vi "Calibration.vi"(0 "Mode":T3, 5 "Calib file":path, 9 "Simulate/Run":T2) -> (14 "Calib const":string[][](array[string]), 16 "Coefficients":dbl[][](array[numeric]) format="%.2f", 19 "Status Out":T1)   [LabVIEW 2014]
uses:
  Anemometry Sub Vis/Calibration/Calib_mode.ctl
  Anemometry Sub Vis/Controls/User_Specific_mode.ctl
  Anemometry Sub Vis/Gen Trav/Multi_Run_Status.ctl
  Anemometry Sub Vis/Controls/Post_Process.ctl
  Anemometry Sub Vis/File/Setup_Filetype.ctl
  Anemometry Sub Vis/Controls/Setup.ctl
  Anemometry Sub Vis/Controls/Save_Data.ctl
  Anemometry Sub Vis/Controls/App_Global.ctl
  <vilib>/Analysis/baseanly.llb/Mean (DBL).vi
  Anemometry Sub Vis/Globals/Calib_global.vi
  Anemometry Sub Vis/Globals/Meas_global.vi
  Anemometry Sub Vis/Acquisition/PWA/PWAtasksGLOBAL.vi
  <vilib>/Analysis/NI_AALBase.lvlib
panel:
  in  "-ve Ref Values":bool
  out "String":string
  in  "polynomial order":i32=2 min=1 max=3 step=1
  out "Ref velocity":dbl[](array[numeric])=[2.4275346736, 2.4395664609, 2.453235235, 2.4247395837, 2.4277603784, 2.41169823, 2.4254144559, 2.424896502176921] format="%.3f"
  out "labels":string[](array[string])=["XW1 Volt", "XW2 Volt", "Entered Val", "Selector"]
  in  "Point selector 3":cluster{"Y":dbl, "X":dbl, "t/f":bool}[](array[cluster]) {"X" format="%#.2g"; "Y" format="%#.3f"}
  in  "n":dbl=0.45 format="%.4f"
  in  "Fixed n":bool=TRUE
  out "Sample of input signals":dbl[][](graph)
  in  "Sampling speeds":T4={"Samples/ch"=600, "Sample Rate/ch (Hz)"=100.0} {"Sample Rate/ch (Hz)" min=0; "Samples/ch" min=0 step=1}
  out "Calibration plot":cluster{cluster{dbl, dbl}[]}[](graph)
  in  "Point selector 4":T5(array[cluster]) {"Y2" format="%#.2f"; "X" format="%#.3f"; "Y" format="%#.2f"}
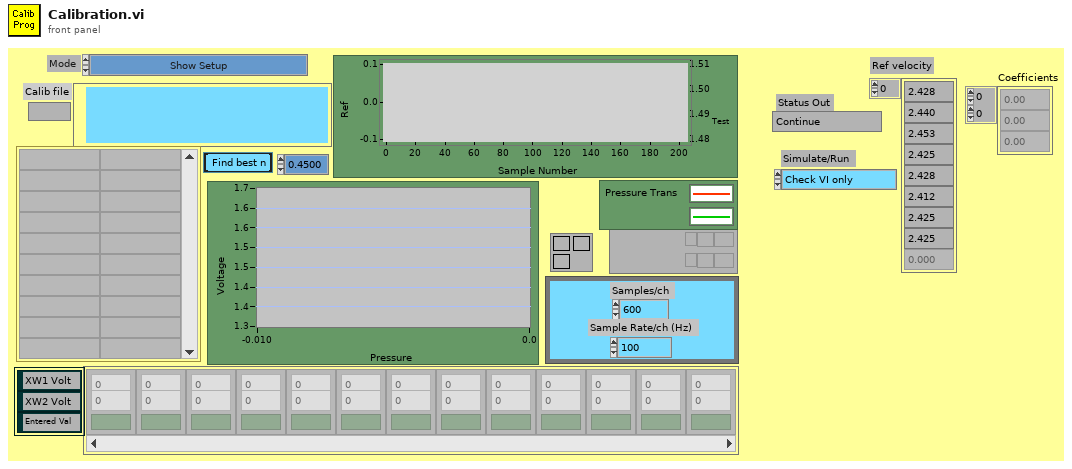
[diagram p1: front panel]
types:
  T1 = typedef "Multi_Run_Status.ctl" = enum16{"Continue", "Jump to Next Point", "Jump to Next Row", "Jump To Fall Back", "Terminate Run"}
  T2 = typedef "User_Specific_mode.ctl" = enum16{"Check VI only", "Run VI"}
  T3 = typedef "Calib_mode.ctl" = enum16{"Show Setup", "Take a New Calibration Point", "Refit Curve", "Setup Front Panel"}
  T4 = cluster{"Samples/ch":i32, "Sample Rate/ch (Hz)":sgl}
  T5 = cluster{"Y":dbl, "Y2":dbl, "X":dbl, "t/f":bool}[]
  T6 = typedef "Post_Process.ctl" = enum16{"Take New Data", "Post Process Raw Data File"}
  T7 = typedef "Setup_Filetype.ctl" = enum16{"Measurement Setups", "Calibration Setups", "General", "Results File Plotter Setups", "Speed Calib Tweaks"}
  T8 = typedef "Save_Data.ctl" = enum16{"Save No Data", "Save Data"}
  T9 = typedef "Setup.ctl" = enum16{"Run Program", "Show Setup", "Save Current Setup", "Setup Front Panel"}
  T10 = typedef "App_Global.ctl" = enum16{"Read Global", "Write to Global", "Initialise Array"}
  T11 = enum32{"existing file", "new file", "new or existing file", "existing dir", "new dir", "new or existing dir", "existing file (use LLBs)", "new file (use LLBs)", "new or existing file (use LLBs)", "new or existing file or directory (use LLBs)"}
  T12 = cluster{"Samples /ch":i32, "Sampling Rate /ch (Hz)":sgl}
  T13 = typedef "Cal_Inst_type.ctl" = enum16{"Propeller anemometer", "Pressure Transducer", "Hot wire", "Cross wire velocity", "Cross wire angle", "Generic Linear", "Generic Polynomial", "Generic BackPoly", "Fast FID", "Thermocouple", "Cold wire", "Pulsed Wire"}
  T14 = typedef "Ref_Inst_type.ctl" = enum16{"Propellor anemometer", "Pressure Transducer", "Raw voltage", "Pitot-static tube", "Preston tube", "Generic Linear", "Generic Polynomial", "Thermocouple", "LDA", "Enter Value", "ADAM Channel"}
  T15 = cluster{"2nd Ref type":T14, "2nd inst present":bool}
  T16 = typedef "Analysis_info_cluster.ctl" = cluster{"Colour":u32, "Inst type":T17, "Inst name":string, "Symbol":string, "Code name":string, "Extra Info":string, "Inst Array":T18, "Extra Titles":string[], "Extra Values":string[], "U":dbl, "u^2":dbl, "u^3":dbl, "u^4":dbl, "Skew_u":dbl, "Kurt_u":dbl, "Sd Error in Mean":dbl, "% u'/U":dbl, "X":dbl, "Y":dbl, "Z":dbl, "Timescale integral to 25%":dbl, "Sd Error in Variance":dbl, "Calib File":path, "Calib Constants":dbl[], "Output Position":bool, "Full Stats":bool, "Av Sampling Rate":dbl, "Av No of Samples":dbl, "Total Meas Time (s)":dbl, "ADAM Ch Name":string}
  T17 = typedef "Inst_type.ctl" = enum16{"Propeller anemometer", "Raw voltage", "Pressure Transducer", "Pitot-static tube", "Preston tube", "Hot wire", "Cross wire 1", "Cross wire 2", "Generic Linear", "Generic Polynomial", "Generic BackPoly", "Fast FID", "Thermocouple", "Cold wire", "Pulsed Wire", "LDA Vel", "LDA Tran time", "LDA Arr time", "Microphone"}
  T18 = typedef "Instrument_Array.ctl" = enum16{"PWA", "LDA", "Analogue"}
  T19 = typedef "Time_Trace_Cluster.ctl" = cluster{"Weighting":dbl[], "Time (s)":dbl[], "Voltage":dbl[], "Eng Values":dbl[]}
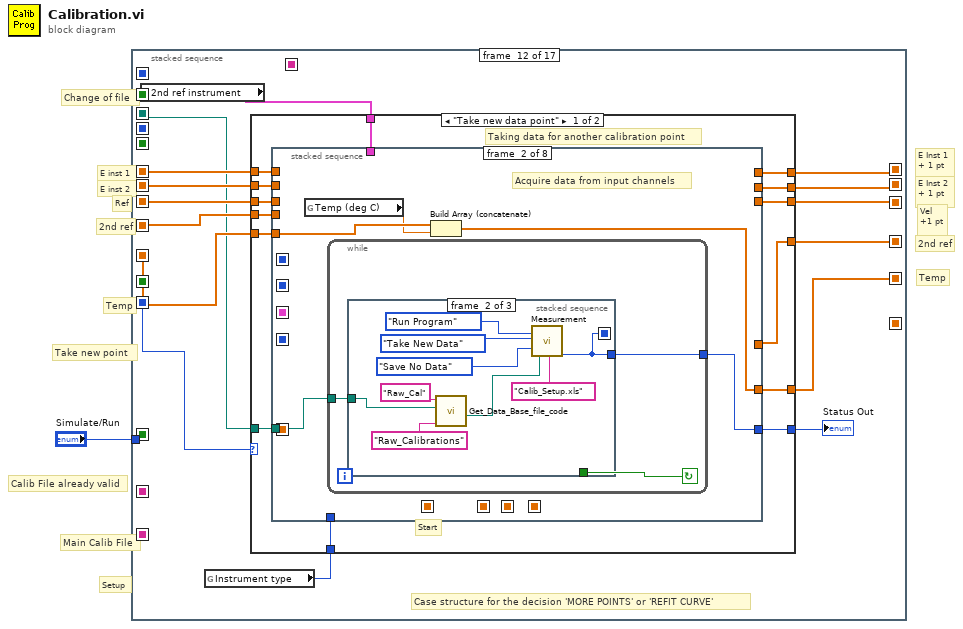
[diagram p0: block diagram]
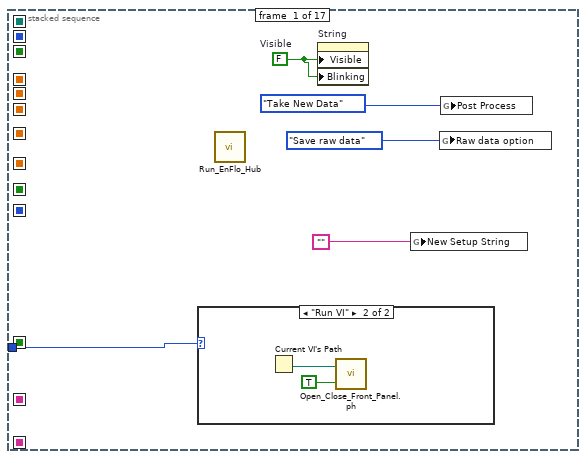
[diagram p2: hidden frame]
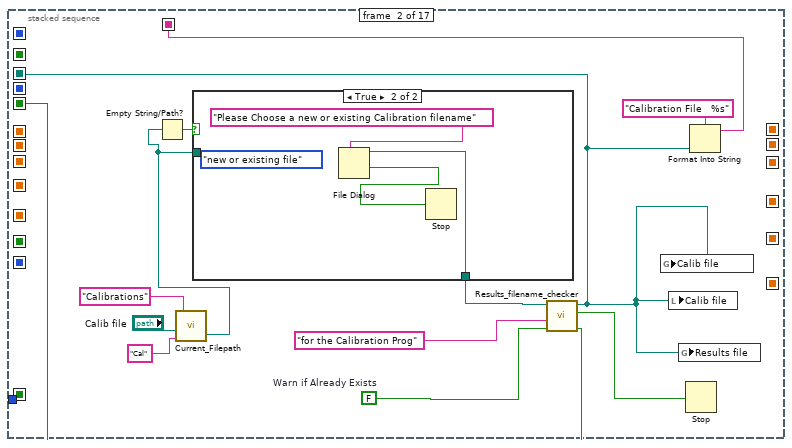
[diagram p4: hidden frame]
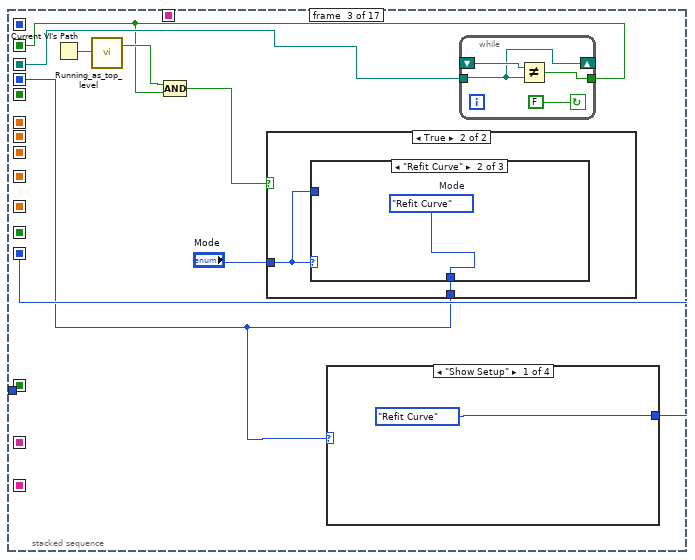
[diagram p6: hidden frame]
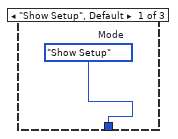
[diagram p8: hidden frame]
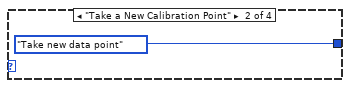
[diagram p10: hidden frame]
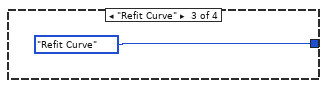
[diagram p11: hidden frame]
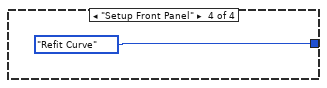
[diagram p12: hidden frame]
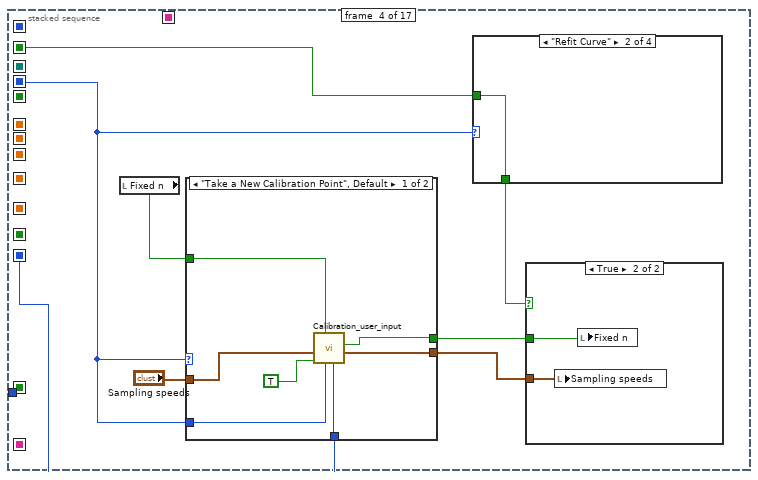
[diagram p13: hidden frame]
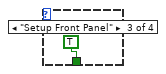
[diagram p15: hidden frame]
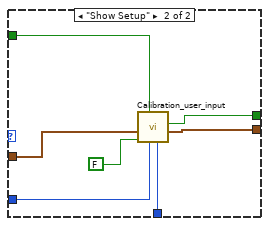
[diagram p18: hidden frame]
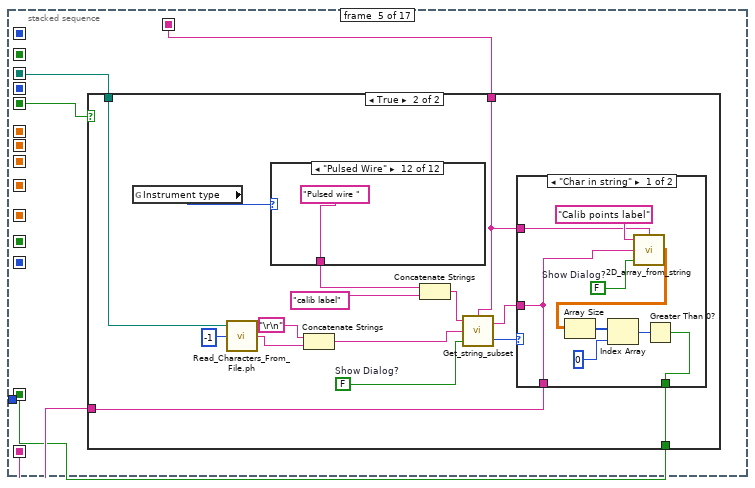
[diagram p19: hidden frame]
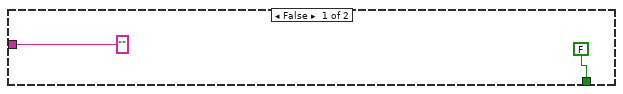
[diagram p20: hidden frame]
diagram:
  # "Change of file"
  # "Take new point"
  # "Calib File already valid"
  # "Main Calib File"
  # "Temp"
  # "Temp"
  # "Setup"
  # "E inst 1"
  # "Ref"
  # "E Inst 1\n+ 1 pt"
  # "Vel\n+1 pt"
  # "E inst 2"
  # "E Inst 2\n+ 1 pt"
  # "2nd ref"
  # "2nd ref"
  n1 = stacked-sequence {
    seq-local: [_ _ _ _ _ _ _ _ _ _ _ w490 _ _ _ _ _] -> [_ _ _ _ _ _ _ _ _ _ _ _ w690 _ _ _ _]
    seq-local: [_ _ _ _ _ _ _ _ _ _ _ w489 _ _ _ _ _] -> [_ _ _ _ _ _ _ _ _ _ _ _ w693 _ _ w756 _]
    seq-local: [_ _ _ _ _ _ _ w377 _ _ _ _ _ _ _ _ _] -> [_ _ _ _ _ _ _ _ _ _ _ w492 _ _ _ _ _]
    seq-local: [_ _ _ _ _ _ _ w376 _ _ _ _ _ _ _ _ _] -> [_ _ _ _ _ _ _ _ _ _ _ w491 _ _ _ _ _]
    seq-local: [_ _ _ _ _ _ _ w375 _ _ _ _ _ _ _ _ _] -> [_ _ _ _ _ _ _ _ _ _ _ w487 _ _ _ _ _]
    seq-local: [_ _ _ _ _ _ _ _ _ _ _ w488 _ _ _ _ _] -> [_ _ _ _ _ _ _ _ _ _ _ _ w692 _ _ _ _]
    seq-local: [_ _ _ _ _ _ _ w374 _ _ _ _ _ _ _ _ _] -> [_ _ _ _ _ _ _ _ _ _ _ w486 _ _ _ _ _]
    seq-local: [_ _ _ _ _ _ _ _ _ _ _ w485 _ _ _ _ _] -> [_ _ _ _ _ _ _ _ _ _ _ _ w687 _ _ _ _]
    seq-local: [_ _ _ _ w79 _ _ _ _ _ _ _ _ _ _ _ _] -> [_ _ _ _ _ _ _ w363 _ _ _ _ _ _ _ _ _]
    seq-local: [_ _ _ _ w80 _ _ _ _ _ _ _ _ _ _ _ _] -> [_ _ _ _ _ _ _ w364 _ _ _ _ _ _ _ _ _]
    seq-local: [_ _ _ _ _ _ _ _ _ _ w465 _ _ _ _ _ _] -> [_ _ _ _ _ _ _ _ _ _ _ _ _ _ w734 _ _]
    seq-local: [_ _ _ _ _ _ _ _ _ _ _ w483 _ _ _ _ _] -> [_ _ _ _ _ _ _ _ _ _ _ _ w691 _ _ _ _]
    seq-local: [_ _ _ _ _ _ _ w373 _ _ _ _ _ _ _ _ _] -> [_ _ _ _ _ _ _ _ _ _ _ w482 _ _ _ _ _]
    seq-local: [_ w14 _ _ _ _ _ _ _ _ _ _ _ _ _ _ _] -> [_ _ w30 _ w78 _ _ _ _ _ w466 w480 _ w716 w743 w757 _]
    seq-local: [_ w19 _ _ _ _ _ _ _ _ _ _ _ _ _ _ _] -> [_ _ _ _ w77 _ _ _ w406 _ _ _ _ _ _ _ _]
    seq-local: [_ _ w33 _ _ _ _ _ _ _ _ _ _ _ _ _ _] -> [_ _ _ w51 _ _ _ _ _ _ _ w479 _ _ _ w758 _]
    seq-local: [_ _ w26 _ _ _ _ _ _ _ _ _ _ _ _ _ _] -> [_ _ _ w50 _ _ _ _ _ w423 _ _ _ _ _ _ w800]
    seq-local: [_ _ _ _ _ _ _ w365 _ _ _ _ _ _ _ _ _] -> [_ _ _ _ _ _ _ _ w404 _ _ _ _ _ _ _ _]
    seq-local: [_ _ _ _ _ _ _ _ _ _ _ _ w688 _ _ _ _] -> [_ _ _ _ _ _ _ _ _ _ _ _ _ w700 _ _ _]
    seq-local: [_ _ _ _ _ _ _ _ _ _ _ _ w686 _ _ _ _] -> [_ _ _ _ _ _ _ _ _ _ _ _ _ w715 _ _ _]
    seq-local: [_ _ w29 _ _ _ _ _ _ _ _ _ _ _ _ _ _] -> [_ _ _ w48 _ _ _ _ w403 _ _ _ _ _ _ _ _]
    seq-local: [_ w13 _ _ _ _ _ _ _ _ _ _ _ _ _ _ _] -> [_ _ _ _ w76 _ _ w358 _ _ _ _ _ _ _ _ _]
    tunnel: "Simulate/Run" -> [w5 _ _ _ _ _ _ _ _ _ _ _ _ _ _ _ _]
    frame #0 {
      w3 = FALSE  # Visible
      n2 = case shown="\"Run VI\"" w5 {
        frame "Check VI only" {
        }
        frame "Run VI" {
          n3 = Current VI's Path() -> (path=w7:path)
          n4 = call "Open_Close_Front_Panel.ph.vi"("Front Panel Window:Open"=TRUE, "VI path"=w7) -> ()  [unwired: 2 out]
        }
      }
      n5 = call "Run_EnFlo_Hub.vi"() -> ()  [unwired: 8 out]
      n6 = property on="String" class="Str"("Visible"=w3, "Blinking"=w3) -> ()  [unwired: 2 in, 2 out]
      n7 = global write "Calib_global.vi" "New Setup String"("") -> ()
      n8 = global write "Meas_global.vi" "Raw data option"(enum16{"Save raw data", "Raw data not saved"}."Save raw data" ("Raw data option")) -> ()
      n9 = global write "Meas_global.vi" "Post Process"(Post_Process."Take New Data" ("Post Process")) -> ()
    }
    frame #1 {
      w20 = FALSE  # Warn if Already Exists
      n10 = call "Current_Filepath.vi"("Short_Name"="Cal" ("Data Type"), "Filename in"="Calib file", "Data Type"="Calibrations") -> ("Filename Out"=w11:path)  [unwired: 1 in, 1 out]
      n11 = Empty String/Path?(string/path=w11) -> (empty?=w16:bool)
      n12 = case shown="True" w16 {
        tunnel: w11 -> [w22 _]
        tunnel: [w22 w24] -> w18
        frame False {
        }
        frame True {
          (unwired) T11."new or existing file" ("select mode (2)")
          n13 = File Dialog(7:"Please Choose a new or existing Calibration filename" ("Promp if not found")) -> (1:w23:bool, 3:w24:path)  [unwired: 1 in, 7 out]
          n14 = Stop(stop? (T)=w23) -> ()
        }
      }
      n15 = call "Results_filename_checker.vi"("Warn if Already Exists"=w20, "Comment"="for the Calibration Prog", "Results file"=w18) -> ("exists?"=w19:bool, "cancelled"=w17:bool, "Results file output"=w14:path)  [unwired: 2 in, 1 out]
      n16 = global write "Calib_global.vi" "Calib file"(w14) -> ()
      n17 = local write "Calib file"(w14) -> ()
      n18 = global write "Meas_global.vi" "Results file"(w14) -> ()
      n19 = Stop(stop? (T)=w17) -> ()
      n20 = Format Into String(format string="Calibration File   %s", w14) -> (resulting string=w13:string)  [unwired: 2 in, 1 out]
    }
    frame #2 {
      n21 = Current VI's Path() -> (path=w32:path)
      n22 = call "Running_as_top_level.vi"("Vi path name"=w32) -> ("Top Level"=w31:bool)  [unwired: 1 out]
      n23 = while {
        shift-right: [w42] -> _
        shift-left: _ -> [w43]
        tunnel: w30 -> [w42]
        tunnel: [w41] -> w29
        stop <- FALSE continue-if-true
        n24 = Not Equal?(x=w43, y=w42) -> (x != y?=w41:bool)
      }
      n25 = Compound Arithmetic op=AND(w31, w29) -> (w28:bool)
      n26 = case shown="True" w28 {
        tunnel: "Mode" -> [w34 w35]
        tunnel: [w34 w36] -> w26
        frame False {
        }
        frame True {
          n27 = case shown="\"Refit Curve\"" w35 {
            tunnel: [w37 w38 w39] -> w36
            tunnel: w35 -> [_ _ w39]
            frame "Show Setup", Default {
              w37 = Calib_mode."Show Setup"  # Mode
            }
            frame "Refit Curve" {
              w38 = Calib_mode."Refit Curve"  # Mode
            }
            frame "Setup Front Panel" {
            }
          }
        }
      }
      n28 = case shown="\"Show Setup\"" w26 {
        tunnel: [enum16{"Take new data point", "Refit Curve"}."Refit Curve" ("data mode") enum16{"Take new data point", "Refit Curve"}."Take new data point" ("data mode") enum16{"Take new data point", "Refit Curve"}."Refit Curve" ("data mode") enum16{"Take new data point", "Refit Curve"}."Refit Curve" ("data mode")] -> w33
        frame "Show Setup" {
        }
        frame "Take a New Calibration Point" {
        }
        frame "Refit Curve" {
        }
        frame "Setup Front Panel" {
        }
      }
    }
    frame #3 {
      n29 = local read "Fixed n"() -> (w53:bool)
      n30 = case shown="\"Take a New Calibration Point\", Default" w50 {
        tunnel: "Sampling speeds" -> [w68 w75]
        tunnel: w50 -> [w66 w73]
        tunnel: w51 -> [w65 w72]
        tunnel: [w64 w71] -> w54
        tunnel: w53 -> [w62 w70]
        tunnel: [w63 w69] -> w52
        frame "Take a New Calibration Point", Default {
          n31 = call "Calibration_user_input.vi"("data mode"=w65, "Mode"=w66, "Fixed n"=w62, "OK"=TRUE, "Sampling speeds"=w68) -> ("Sampling speeds Output"=w64:T12, "Fixed n out"=w63:bool)  [unwired: 2 in, 3 out]
        }
        frame "Show Setup" {
          n32 = call "Calibration_user_input.vi"("data mode"=w72, "Mode"=w73, "Fixed n"=w70, "OK"=FALSE, "Sampling speeds"=w75) -> ("Sampling speeds Output"=w71:T12, "Fixed n out"=w69:bool)  [unwired: 5 out]
        }
      }
      n33 = case shown="\"Refit Curve\"" w50 {
        tunnel: [w56 w57 TRUE w59] -> w49
        tunnel: w48 -> [w56 w57 _ w59]
        frame "Show Setup" {
        }
        frame "Refit Curve" {
        }
        frame "Setup Front Panel" {
        }
        frame "Take a New Calibration Point" {
        }
      }
      n34 = case shown="True" w49 {
        tunnel: w54 -> [_ w61]
        tunnel: w52 -> [_ w60]
        frame False {
        }
        frame True {
          n35 = local write "Sampling speeds"(w61) -> ()
          n36 = local write "Fixed n"(w60) -> ()
        }
      }
    }
    frame #4 {
      n37 = case shown="True" w77 {
        tunnel: ["" ("Output string") w97] -> w80
        tunnel: [FALSE w96] -> w79
        tunnel: w78 -> [_ w88]
        tunnel: w76 -> [_ w83]
        frame False {
        }
        frame True {
          w87 = FALSE  # Show Dialog?
          n38 = global read "Calib_global.vi" "Instrument type"() -> (w91:T13)
          n39 = call "Read_Characters_From_File.ph.vi"("file path (dialog if empty)"=w88, "number of characters (all:-1)"=-1) -> ("character string"=w85:string)  [unwired: 7 out]
          n40 = case shown="\"Pulsed Wire\"" w91 {
            tunnel: ["Prop " "Mano " "HW " "Cross wire velocity " "Cross wire angle " "Generic Inst " "Generic Polynomial " "Generic BackPoly " "Fast FID " "Thermocouple " "Cold wire " "Pulsed wire "] -> w92
            frame "Propeller anemometer" {
            }
            frame "Pressure Transducer" {
            }
            frame "Hot wire" {
            }
            frame "Cross wire velocity" {
            }
            frame "Cross wire angle" {
            }
            frame "Generic Linear" {
            }
            frame "Generic Polynomial" {
            }
            frame "Generic BackPoly" {
            }
            frame "Fast FID" {
            }
            frame "Thermocouple" {
            }
            frame "Cold wire" {
            }
            frame "Pulsed Wire" {
            }
          }
          n41 = Concatenate Strings("\r\n", w85) -> (w84:string)
          n42 = Concatenate Strings(w92, "calib label") -> (w93:string)
          n43 = call "Get_string_subset.vi"("String Name"=w83, "Show Dialog?"=w87, "String to split"=w84, "File Label"=w93) -> ("Status"=w90:enum16{"Char in string", "Char not in string"}, "Output string"=w89:string)
          n44 = case shown="\"Char in string\"" w90 {
            tunnel: w89 -> [w116 _]
            tunnel: [w116 ""] -> w97
            tunnel: [w111 FALSE] -> w96
            tunnel: w83 -> [w110 _]
            frame "Char in string" {
              w117 = FALSE  # Show Dialog?
              n45 = call "2D_array_from_string.vi"("String Name"=w110, "Show Dialog?"=w117, "Input string"=w116, "Array title"="Calib points label") -> ("2D data array"=w115:dbl[][])
              n46 = Array Size(array=w115) -> (size(s)=w114:i32[])
              n47 = Index Array(array=w114, index=0 ("Index")) -> (element=w112:i32)
              n48 = Greater Than 0?(x=w112) -> (x > 0?=w111:bool)
            }
            frame "Char not in string" {
            }
          }
        }
      }
    }
    frame #5 {
      w123 = ""
      n49 = global read "Calib_global.vi" "2nd ref instrument"() -> (w130:T15)
      n50 = global read "Calib_global.vi" "Ref Instrument type"() -> (w131:T14)
      n51 = Unbundle By Name(w130) -> ("2nd Ref type"=w128:T14, "2nd inst present"=w129:bool)
      n52 = global read "Calib_global.vi" "Instrument type"() -> (w134:T13)
      n53 = case shown="\"Propellor anemometer\"" w131 {
        tunnel: [w160 w163 w167 w169 w172 w175 w178 w181 w184 string[] [] string[] []] -> w127
        tunnel: [FALSE FALSE FALSE FALSE TRUE FALSE FALSE FALSE FALSE FALSE FALSE] -> w122
        frame "Propellor anemometer" {
          n54 = Build Array("Prop Velocity") -> (w160:string[])
        }
        frame "Pressure Transducer" {
          n55 = Build Array("Pressure Trans") -> (w163:string[])
        }
        frame "Raw voltage" {
          n56 = Build Array("Raw Voltage") -> (w167:string[])
        }
        frame "Pitot-static tube" {
          n57 = Build Array("Pitot Vel") -> (w169:string[])
        }
        frame "Preston tube" {
          n58 = Build Array("Shear stress") -> (w172:string[])
        }
        frame "Generic Linear" {
          n59 = Build Array("Gen Lin") -> (w175:string[])
        }
        frame "Generic Polynomial" {
          n60 = Build Array("Gen Poly") -> (w178:string[])
        }
        frame "Thermocouple" {
          n61 = Build Array("Thermo") -> (w181:string[])
        }
        frame "LDA" {
          n62 = Build Array("LDA Vel") -> (w184:string[])
        }
        frame "Enter Value" {
        }
        frame "ADAM Channel" {
        }
      }
      n63 = case shown="True" w129 {
        tunnel: w128 -> [_ w137]
        tunnel: [w136 w138] -> w125
        tunnel: w127 -> [w136 _]
        frame False {
        }
        frame True {
          n64 = case shown="\"Propellor anemometer\"" w137 {
            tunnel: [w139 w141 w144 w145 w147 w149 w151 w153 w155 string[] [] string[] []] -> w138
            frame "Propellor anemometer" {
              n65 = Build Array("Prop Velocity") -> (w139:string[])
            }
            frame "Pressure Transducer" {
              n66 = Build Array("Pressure Trans") -> (w141:string[])
            }
            frame "Raw voltage" {
              n67 = Build Array("Raw Voltage") -> (w144:string[])
            }
            frame "Pitot-static tube" {
              n68 = Build Array("Pitot Vel") -> (w145:string[])
            }
            frame "Preston tube" {
              n69 = Build Array("Shear stress") -> (w147:string[])
            }
            frame "Generic Linear" {
              n70 = Build Array("Gen Lin") -> (w149:string[])
            }
            frame "Generic Polynomial" {
              n71 = Build Array("Gen Poly") -> (w151:string[])
            }
            frame "Thermocouple" {
              n72 = Build Array("Thermo") -> (w153:string[])
            }
            frame "LDA" {
              n73 = Build Array("LDA Vel") -> (w155:string[])
            }
            frame "Enter Value" {
            }
            frame "ADAM Channel" {
            }
          }
        }
      }
      n74 = case shown="\"Pulsed Wire\"" w134 {
        tunnel: [w194 w198 w202 w206 w211 w216 w220 w224 w228 w232 w236 w241] -> w124
        tunnel: [FALSE FALSE FALSE FALSE FALSE FALSE TRUE TRUE FALSE FALSE TRUE TRUE] -> w126
        tunnel: [w192 w196 w200 w204 w209 w214 w218 w222 w226 w230 w234 FALSE] -> w121
        tunnel: w122 -> [w192 w196 w200 w204 w209 w214 w218 w222 w226 w230 w234 _]
        frame "Propeller anemometer" {
          n75 = Build Array("Prop Voltage") -> (w194:string[])
        }
        frame "Pressure Transducer" {
          n76 = Build Array("Pressure Trans") -> (w198:string[])
        }
        frame "Hot wire" {
          n77 = Build Array("HW Voltage") -> (w202:string[])
        }
        frame "Cross wire velocity" {
          n78 = Build Array("XW1 Voltage", "XW2 Voltage") -> (w206:string[])
        }
        frame "Cross wire angle" {
          n79 = Build Array("XW1 Voltage", "XW2 Voltage") -> (w211:string[])
        }
        frame "Generic Linear" {
          n80 = Build Array("Generic Voltage") -> (w216:string[])
        }
        frame "Generic Polynomial" {
          n81 = Build Array("Generic Voltage") -> (w220:string[])
        }
        frame "Generic BackPoly" {
          n82 = Build Array("Generic Voltage") -> (w224:string[])
        }
        frame "Fast FID" {
          n83 = Build Array("FF Voltage") -> (w228:string[])
        }
        frame "Thermocouple" {
          n84 = Build Array("Thermo Voltage") -> (w232:string[])
        }
        frame "Cold wire" {
          n85 = Build Array("CW Voltage") -> (w236:string[])
        }
        frame "Pulsed Wire" {
          n86 = local write "polynomial order"(3 ("polynomial order")) -> ()
          n87 = Build Array("PWA 1/TOF") -> (w241:string[])
        }
      }
      n88 = property on="polynomial order" class="DigNum (strict)"("Visible"=w126) -> ()  [unwired: 2 in, 2 out]
      n89 = Build Array (concatenate)(w125, w124, w123, w123, w123) -> (w132:string[])
      n90 = for {
        N: 3 -> [_]
        tunnel: w132 -> [w190] mode=indexing
        i -> [w191]
        n91 = property on="Sample of input signals" class="WFGraph (strict)"("Active Plot"=w191, "Plot.Plot Name"=w190) -> ()  [unwired: 2 in, 2 out]
      }
      n92 = case shown="False" w121 {
        frame False {
          n93 = local write "-ve Ref Values"(FALSE ("-ve Ref Values")) -> ()
        }
        frame True {
        }
      }
      n94 = property on="-ve Ref Values" class="Bool (strict)"("Visible"=w121) -> ()  [unwired: 2 in, 2 out]
    }
    frame #6 {
      n95 = global read "Calib_global.vi" "Instrument type"() -> (w246:T13)
      n96 = global read "Calib_global.vi" "Ref Instrument type"() -> (w245:T14)
      n97 = case shown="\"Propellor anemometer\"" w245 {
        tunnel: ["Prop Vel" "Pressure" "Voltage" "Pitot Vel" "Shear stress" "Generic Linear" "Generic Poly" "Thermo T" "LDA Vel" "Entered Val" "ADAM Channel"] -> w248
        frame "Propellor anemometer" {
        }
        frame "Pressure Transducer" {
        }
        frame "Raw voltage" {
        }
        frame "Pitot-static tube" {
        }
        frame "Preston tube" {
        }
        frame "Generic Linear" {
        }
        frame "Generic Polynomial" {
        }
        frame "Thermocouple" {
        }
        frame "LDA" {
        }
        frame "Enter Value" {
        }
        frame "ADAM Channel" {
        }
      }
      n98 = case shown="\"Pulsed Wire\"" w246 {
        tunnel: [FALSE FALSE TRUE TRUE TRUE FALSE FALSE FALSE FALSE FALSE FALSE FALSE] -> w251
        tunnel: [TRUE TRUE TRUE FALSE FALSE TRUE TRUE TRUE TRUE TRUE TRUE TRUE] -> w250
        tunnel: [FALSE FALSE FALSE TRUE TRUE FALSE FALSE FALSE FALSE FALSE FALSE FALSE] -> w249
        tunnel: w248 -> [w264 w271 w280 w290 w300 w310 w316 w323 w330 w338 w344 w351]
        tunnel: [w267 w274 w283 w293 w303 w312 w319 w326 w333 w340 w347 w354] -> w247
        tunnel: "Selector" -> [w266 w273 w282 w292 w302 w309 w318 w325 w332 w337 w346 w353]
        tunnel: [w265 w272 "E^2" "XW Volt^2" "Y" w311 w316 w324 w330 w339 w344 w351] -> w243
        tunnel: [w264 w271 w278 w288 "X" w310 w317 w323 w331 w338 w345 w352] -> w244
        frame "Propeller anemometer" {
          w265 = "Prop Volt"
          n99 = Build Array(w265, w264, w266) -> (w267:string[])
        }
        frame "Pressure Transducer" {
          w272 = "Voltage"
          n100 = Build Array(w272, w271, w273) -> (w274:string[])
        }
        frame "Hot wire" {
          n101 = Build Array("HW Volt", w280, w282) -> (w283:string[])
          n102 = Concatenate Strings(w280, "^n") -> (w278:string)
        }
        frame "Cross wire velocity" {
          n103 = Build Array("XW1 Volt", "XW2 Volt", w290, w292) -> (w293:string[])
          n104 = Concatenate Strings(w290, "^n") -> (w288:string)
        }
        frame "Cross wire angle" {
          n105 = Build Array("XW1 Volt", "XW2 Volt", w300, w302) -> (w303:string[])
        }
        frame "Generic Linear" {
          w311 = "Gen Volt"
          n106 = Build Array(w311, w310, w309) -> (w312:string[])
        }
        frame "Generic Polynomial" {
          w317 = "Gen Volt"
          n107 = Build Array(w317, w316, w318) -> (w319:string[])
        }
        frame "Generic BackPoly" {
          w324 = "Gen Volt"
          n108 = Build Array(w323, w324, w325) -> (w326:string[])
        }
        frame "Fast FID" {
          w331 = "FF Volt"
          n109 = Build Array(w331, w330, w332) -> (w333:string[])
        }
        frame "Thermocouple" {
          w339 = "Thermo Volt"
          n110 = Build Array(w339, w338, w337) -> (w340:string[])
        }
        frame "Cold wire" {
          w345 = "CW Volt"
          n111 = Build Array(w345, w344, w346) -> (w347:string[])
        }
        frame "Pulsed Wire" {
          w352 = "1/TOF"
          n112 = Build Array(w352, w351, w353) -> (w354:string[])
        }
      }
      "labels" <- w247
      n113 = property on="n" class="DigNum (strict)"("Visible"=w251) -> ()  [unwired: 2 in, 2 out]
      n114 = property on="Fixed n" class="Bool (strict)"("Visible"=w251) -> ()  [unwired: 2 in, 2 out]
      n115 = property on="Calibration plot" class="XYGraph (strict)"("X Scale.Name Label.Text"=w244, "Y Scale.Name Label.Text"=w243) -> ()  [unwired: 2 in, 2 out]
      n116 = property on="Point selector 3" class="Arr (strict)"("Visible"=w250) -> ()  [unwired: 2 in, 2 out]
      n117 = property on="Point selector 4" class="Arr (strict)"("Visible"=w249) -> ()  [unwired: 2 in, 2 out]
    }
    frame #7 {
      # "Case structure to read previous calibration points if required"
      n118 = global read "Calib_global.vi" "Calibration Points"() -> (w362:dbl[])
      n119 = case shown="True" w363 {
        tunnel: w364 -> [_ w397]
        tunnel: [w389 w394] -> w361
        tunnel: w362 -> [w390 w393]
        tunnel: w358 -> [_ w391]
        frame False {
          n120 = Build Array(w390) -> (w389:dbl[][])
        }
        frame True {
          w396 = FALSE  # Show Dialog?
          n121 = Array Size(array=w393) -> (size(s)=w392:i32)
          n122 = call "2D_array_from_string.vi"("String Name"=w391, "Show Dialog?"=w396, "Input string"=w397, "Array title"="Calib points label") -> ("2D data array"=w395:dbl[][])
          n123 = case shown="0" w392 {
            tunnel: w395 -> [w399 w402]
            tunnel: [w399 w401] -> w394
            tunnel: w393 -> [_ w400]
            frame 0 {
            }
            frame 1, Default {
              n124 = Build Array (concatenate)(w402, w400) -> (w401:dbl[][])
            }
          }
        }
      }
      n125 = for {
        tunnel: w361 -> [w379] mode=indexing
        shift-right: [w378] -> w359
        shift-left: dbl[][] [] -> [w380]
        n126 = Array Subset(array=w379, length=2) -> (w383:dbl[])  [unwired: 1 in]
        n127 = Not A Number/Path/Refnum?(number/path/refnum=w383) -> (NaN/Path/Refnum?=w382:bool[])
        n128 = Or Array Elements(Boolean array=w382) -> (logical OR=w381:bool)
        n129 = case shown="False" w381 {
          tunnel: w380 -> [w387 w388]
          tunnel: w379 -> [w386 _]
          tunnel: [w385 w388] -> w378
          frame False {
            n130 = Build Array (concatenate)(w387, w386) -> (w385:dbl[][])
          }
          frame True {
          }
        }
      }
      n131 = Index Array(array=w359, index (col)=0) -> (element=w376:dbl[])  [unwired: 1 in]
      n132 = Index Array(array=w359, index (col)=1) -> (element=w377:dbl[])  [unwired: 1 in]
      n133 = Index Array(array=w359, index (col)=2) -> (element=w375:dbl[])  [unwired: 1 in]
      n134 = Index Array(array=w359, index (col)=3) -> (element=w374:dbl[])  [unwired: 1 in]
      n135 = Index Array(array=w359, index (col)=4) -> (element=w373:dbl[])  [unwired: 1 in]
      n136 = Index Array(array=w359, index (col)=5) -> (element=w366:dbl[])  [unwired: 1 in]
      n137 = Not A Number/Path/Refnum?(number/path/refnum=w366) -> (NaN/Path/Refnum?=w365:bool[])
    }
    frame #8 {
      n138 = And(x=w403, y=w406) -> (x .and. y?=w405:bool)
      n139 = case shown="True" w405 {
        tunnel: w404 -> [_ w407]
        frame False {
        }
        frame True {
          n140 = local read "Point selector 3"() -> (w411:cluster{"Y":dbl, "X":dbl, "t/f":bool}[])
          n141 = local read "Point selector 4"() -> (w408:T5)
          n142 = for {
            tunnel: w411 -> [w419]
            tunnel: [w421] -> w410 mode=indexing
            tunnel: w407 -> [w420] mode=indexing
            i -> [w418]
            n143 = Index Array(array=w419, index=w418) -> (element=w417:cluster{"Y":dbl, "X":dbl, "t/f":bool})
            n144 = Bundle By Name(cluster=w417, "t/f"=w420) -> (w421:cluster{"Y":dbl, "X":dbl, "t/f":bool})
          }
          n145 = for {
            tunnel: w408 -> [w414]
            tunnel: [w416] -> w409 mode=indexing
            tunnel: w407 -> [w415] mode=indexing
            i -> [w413]
            n146 = Index Array(array=w414, index=w413) -> (element=w412:cluster{"Y":dbl, "Y2":dbl, "X":dbl, "t/f":bool})
            n147 = Bundle By Name(cluster=w412, "t/f"=w415) -> (w416:cluster{"Y":dbl, "Y2":dbl, "X":dbl, "t/f":bool})
          }
          n148 = local write "Point selector 3"(w410) -> ()
          n149 = local write "Point selector 4"(w409) -> ()
        }
      }
    }
    frame #9 {
      w426 = "Setup for instrument being calibrated"
      n150 = global read "Calib_global.vi" "Pre Setup String"() -> (w424:string)
      n151 = case shown="\"Show Setup\"" w423 {
        tunnel: w424 -> [w431 w435]
        tunnel: w426 -> [w430 w434]
        tunnel: [w429 w433] -> w425
        tunnel: "Previous Setup String" ("String Name") -> [w428 w432]
        frame "Take a New Calibration Point", Default {
          n152 = call "Get_string_subset.vi"("String Name"=w428, "String to split"=w431, "File Label"=w430) -> ("Output string"=w429:string)  [unwired: 1 in, 1 out]
        }
        frame "Show Setup" {
          n153 = global read "Calib_global.vi" "Instrument type"() -> (w439:T13)
          n154 = call "Get_string_subset.vi"("String Name"=w432, "String to split"=w435, "File Label"=w434) -> ("Status"=w437:enum16{"Char in string", "Char not in string"}, "Output string"=w438:string)  [unwired: 1 in]
          n155 = case shown="\"Char in string\"" w437 {
            tunnel: [w440 w441] -> w436
            tunnel: w438 -> [w440 _]
            tunnel: w435 -> [_ w441]
            frame "Char in string" {
            }
            frame "Char not in string" {
            }
          }
          n156 = case shown="\"Cross wire velocity\"" w439 {
            tunnel: [w443 w445 w448 w451 w454 w456 w458 w460 ""] -> w433
            tunnel: w436 -> [w442 w444 w446 w449 w452 w455 w457 w459 _]
            frame "Propeller anemometer" {
              n157 = call "Propeller_setup.vi"("Setup String"=w442) -> ("Output string"=w443:string)
            }
            frame "Pressure Transducer" {
              n158 = call "Pressure_Transducer_Setup.vi"("Setup String"=w444) -> ("Output string"=w445:string)
            }
            frame "Hot wire" {
              n159 = call "Hot_Wire_Setup.vi"("XW?"=FALSE, "Setup String"=w446) -> ("Output string"=w448:string)
            }
            frame "Cross wire velocity" {
              n160 = call "Hot_Wire_Setup.vi"("XW?"=TRUE, "Setup String"=w449) -> ("Output string"=w451:string)
            }
            frame "Cross wire angle" {
              n161 = call "Hot_Wire_Setup.vi"("XW?"=TRUE, "Setup String"=w452) -> ("Output string"=w454:string)
            }
            frame "Generic Linear" {
              n162 = call "Generic_setup.vi"("Setup String"=w455) -> ("Output String"=w456:string)
            }
            frame "Generic Polynomial" {
              n163 = call "Generic_setup.vi"("Setup String"=w457) -> ("Output String"=w458:string)
            }
            frame "Generic BackPoly" {
              n164 = call "Generic_setup.vi"("Setup String"=w459) -> ("Output String"=w460:string)
            }
            frame "Fast FID", Default {
            }
          }
        }
      }
      n165 = call "Add_label_to_string.vi"("String to write"=w425, "File Label"=w426) -> ("Output string"=w427:string)
      n166 = global write "Calib_global.vi" "Instument setup Info"(w427) -> ()
    }
    frame #10 {
      w467 = TRUE  # Lock File
      w473 = FALSE  # advisory dialog? (display:T)
      w474 = FALSE  # append to file? (new file:F)
      n167 = global read "Calib_global.vi" "Instument setup Info"() -> (w469:string)
      n168 = Path To String(path=w466) -> (string=w468:string)
      n169 = global read "Calib_global.vi" "New Setup String"() -> (w470:string)
      n170 = call "Date_and_Time_to_string.vi"() -> ("Date and time (spreadsheet)"=w476:string)
      n171 = call "Characters_to_string.vi"("Characters to write"=w468, "Label for characters"="Calib filename") -> ("Output string"=w477:string)
      n172 = Concatenate Strings(w476, w477, w470, w469) -> (w465:string)
      n173 = call "Add_label_to_string.vi"("String to write"=w465, "File Label"="Raw data header") -> ("Output string"=w471:string)
      n174 = call "Setup_Filepath.vi"("Setup File Type"=Setup_Filetype."Calibration Setups", "Filename in"="Current_Setup.xls") -> ("Filename Out"=w462:path)  [unwired: 1 out]
      n175 = call "Calib_read_files.vi"() -> ()  [unwired: 1 out]
      n176 = call "Write_Characters_To_File.vi"("file path (dialog if empty)"=w462, "advisory dialog? (display:T)"=w473, "character string"=w471, "append to file? (new file:F)"=w474, "Lock File"=w467) -> ()  [unwired: 4 out]
    }
    frame #11 {
      # "Case structure for the decision 'MORE POINTS' or 'REFIT CURVE'"
      n177 = global read "Calib_global.vi" "2nd ref instrument"() -> (w484:T15)
      n178 = global read "Calib_global.vi" "Instrument type"() -> (w478:T13)
      n179 = case shown="\"Take new data point\"" w479 {
        tunnel: [w503 w685] -> w489
        tunnel: [w504 w681] -> w490
        tunnel: w492 -> [w505 w685]
        tunnel: w491 -> [w506 w681]
        tunnel: [w502 w684] -> w488
        tunnel: w487 -> [w501 w684]
        tunnel: w486 -> [w500 w683]
        tunnel: [w498 w683] -> w485
        tunnel: w484 -> [w499 _]
        tunnel: [w496 w682] -> w483
        tunnel: w482 -> [w497 w682]
        tunnel: w480 -> [w495 _]
        tunnel: [w494 Multi_Run_Status."Continue" ("Status Out")] -> w481
        tunnel: w478 -> [w493 _]
        frame "Take new data point" {
          # "Start"
          # "Taking data for another calibration point"
          n180 = stacked-sequence {
            seq-local: [_ _ _ _ w571 _ _ _] -> [_ _ _ _ _ w589 _ _]
            seq-local: [w510 _ _ _ _ _ _ _] -> [_ _ _ _ w572 w582 _ _]
            seq-local: [_ _ w537 _ _ _ _ _] -> [_ _ _ _ _ _ w618 _]
            seq-local: [_ _ _ _ _ w581 _ _] -> [_ _ _ _ _ _ w617 _]
            seq-local: [_ _ w535 _ _ _ _ _] -> [_ _ _ _ _ w580 w616 _]
            seq-local: [_ _ _ w552 _ _ _ _] -> [_ _ _ _ w567 _ _ _]
            seq-local: [_ _ _ w550 _ _ _ _] -> [_ _ _ _ _ _ w614 _]
            seq-local: [_ _ _ w549 _ _ _ _] -> [_ _ _ _ _ _ w613 _]
            seq-local: [_ _ _ w548 _ _ _ _] -> [_ _ _ _ _ w578 _ _]
            tunnel: w505 -> [_ _ _ _ _ _ w622 _]
            tunnel: [_ _ _ _ w574 _ _ _] -> w504
            tunnel: w506 -> [_ _ _ _ w573 _ _ _]
            tunnel: [_ _ _ _ _ _ w621 _] -> w503
            tunnel: [_ _ _ _ _ _ w620 _] -> w502
            tunnel: w501 -> [_ _ _ _ _ _ w619 _]
            tunnel: w500 -> [_ _ _ _ _ w585 _ _]
            tunnel: [_ _ _ _ _ w584 _ _] -> w498
            tunnel: w499 -> [_ _ _ _ _ w583 _ _]
            tunnel: w497 -> [_ w515 _ _ _ _ _ _]
            tunnel: [_ w514 _ _ _ _ _ _] -> w496
            tunnel: w495 -> [_ w512 _ _ _ _ _ _]
            tunnel: [_ w513 _ _ _ _ _ _] -> w494
            tunnel: w493 -> [_ _ _ w551 _ w579 w615 _]
            frame #0 {
              w507 = TRUE  # Visible
              w508 = "Currently Taking a New Calibration Point"  # String
              n181 = Get Date/Time In Seconds() -> (seconds since 1Jan1904=w509:timestamp)
              n182 = To Double Precision Float(number=w509) -> (double precision float=w510:dbl)
              n183 = property on="String" class="Str"("Visible"=w507, "Blinking"=w507) -> ()  [unwired: 2 in, 2 out]
              "String" <- w508
            }
            frame #1 {
              # "Acquire data from input channels"
              n184 = global read "Calib_global.vi" "Temp (deg C)"() -> (w511:dbl)
              n185 = while {
                tunnel: [w518] -> w513
                tunnel: w512 -> [w517]
                stop <- w516 continue-if-true
                n186 = stacked-sequence {
                  seq-local: [_ w521 _] -> [_ _ w529]
                  tunnel: [_ w521 _] -> w518
                  tunnel: w517 -> [_ w525 _]
                  tunnel: [_ _ w530] -> w516
                  frame #0 {
                    n187 = global write "Meas_global.vi" "Remote control"(TRUE ("Remote control")) -> ()
                  }
                  frame #1 {
                    n188 = call "Get_Data_Base_file_code.vi"("Data Type"="Raw_Calibrations", "Results Filename"=w525, "Short_Name"="Raw_Cal" ("Data Type")) -> ("Raw Data File Name"=w522:path)  [unwired: 1 in, 3 out]
                    n189 = call "Measurement.vi"("setup"=Setup."Run Program", "Post Process"=Post_Process."Take New Data", "File"=Save_Data."Save No Data", "Raw data file"=w522, "Setup filename"="Calib_Setup.xls") -> ("Status Out"=w521:T1)  [unwired: 2 in, 12 out]
                  }
                  frame #2 {
                    n190 = global read "Meas_global.vi" "Repeat Measurement?"() -> (w531:bool)
                    n191 = Equal?(x=w529, y=Multi_Run_Status."Continue" ("Status Out")) -> (x = y?=w532:bool)
                    n192 = And(x=w532, y=w531) -> (x .and. y?=w530:bool)
                  }
                }
              }
              n193 = Build Array (concatenate)(w515, w511) -> (w514:dbl[])
            }
            frame #2 {
              n194 = global read "Meas_global.vi" "Analysis Info cluster"() -> (w537:T16[])
              n195 = global read "Meas_global.vi" "Time Trace"() -> (w534:T19[])
              n196 = for {
                tunnel: w537 -> [w543] mode=indexing
                shift-right: [w540] -> w535
                shift-left: dbl[][] [] -> [w541]
                tunnel: w534 -> [w539] mode=indexing
                n197 = Unbundle By Name(w539) -> ("Eng Values"=w538:dbl[])
                n198 = Unbundle By Name(w543) -> ("Inst Array"=w542:T18)
                n199 = case shown="\"PWA\", Default" w542 {
                  tunnel: w541 -> [w544 w547]
                  tunnel: w538 -> [_ w546]
                  tunnel: [w544 w545] -> w540
                  frame "PWA", Default {
                  }
                  frame "Analogue" {
                    n200 = Build Array (concatenate)(w547, w546) -> (w545:dbl[][])
                  }
                }
              }
              "Sample of input signals" <- w535
            }
            frame #3 {
              n201 = case shown="\"Pulsed Wire\"" w551 {
                tunnel: [0 ("Index in") 1 ("Index in")] -> w552
                tunnel: [w553 w556] -> w550
                tunnel: [w553 w560] -> w549
                tunnel: [w553 w559] -> w548
                frame "Propeller anemometer", Default {
                  w553 = 0.0 ("mean")
                }
                frame "Pulsed Wire" {
                  n202 = global read "PWAtasksGLOBAL.vi" "PWA 1/TOF"() -> (w563:dbl[][])
                  n203 = Index Array(array=w563, index (row)=0) -> (element=w561:dbl[])  [unwired: 1 in]
                  n204 = call "Mean_fr_NaN_data.vi"("Data"=w561) -> ("Mean value"=w556:dbl)  [unwired: 1 out]
                  n205 = Less Than 0?(x=w556) -> (x < 0?=w555:bool)
                  n206 = local write "-ve Ref Values"(w555) -> ()
                  n207 = Multiply(x=w561, y=w561) -> (x*y=w558:dbl[])
                  n208 = call "Mean_fr_NaN_data.vi"("Data"=w558) -> ("Mean value"=w560:dbl)  [unwired: 1 out]
                  n209 = Multiply(x=w561, y=w558) -> (x*y=w557:dbl[])
                  n210 = call "Mean_fr_NaN_data.vi"("Data"=w557) -> ("Mean value"=w559:dbl)  [unwired: 1 out]
                }
              }
            }
            frame #4 {
              # "Adding the velocity value to the array"
              n211 = global read "Calib_global.vi" "ADAM Channel Name"() -> (w565:string)
              n212 = global read "Calib_global.vi" "Ref Instrument type"() -> (w570:T14)
              n213 = call "Get_ref_inst_value.vi"("Ref Instrument type"=w570, "ADAM Channel Name"=w565, "Index in"=w567, "Start time"=w572) -> ("Ref Value"=w569:dbl, "Index out"=w571:i32)  [unwired: 3 in, 7 out]
              n214 = case shown="True" "-ve Ref Values" {
                tunnel: w569 -> [w575 w577]
                tunnel: [w575 w576] -> w568
                frame False {
                }
                frame True {
                  n215 = Negate(x=w577) -> (-x=w576:dbl)
                }
              }
              n216 = Build Array (concatenate)(w573, w568) -> (w574:dbl[])
            }
            frame #5 {
              n217 = Unbundle(w583) -> ("2nd Ref type"=w587:T14, "2nd inst present"=w586:bool)
              n218 = case shown="False" w586 {
                tunnel: w589 -> [w594 w609]
                tunnel: [w592 w610] -> w588
                tunnel: w587 -> [_ w611]
                tunnel: w582 -> [_ w612]
                tunnel: [w594 w608] -> w581
                tunnel: w580 -> [w593 _]
                tunnel: w579 -> [w591 _]
                tunnel: w578 -> [w590 _]
                frame False {
                  n219 = case shown="\"Fast FID\"" w591 {
                    tunnel: w594 -> [_ _ w605 _]
                    tunnel: w593 -> [_ _ w604 _]
                    tunnel: [0.0 ("mean") w596 w602 w606] -> w592
                    tunnel: w590 -> [_ _ _ w606]
                    frame "Propeller anemometer", Default {
                    }
                    frame "Fast FID" {
                      n220 = Build Array("GMU:Source:ppm/%Density") -> (w599:string[])
                      n221 = call "Get_Channel_averages.vi"("Desired Ch Names"=w599, "Averaging time (mins)"=0.2) -> ("number"=w597:dbl[])  [unwired: 1 in, 2 out]
                      n222 = Index Array(array=w597) -> (element=w596:dbl)  [unwired: 1 in]
                    }
                    frame "Generic Polynomial" {
                      n223 = Index Array(array=w604, index (row)=w605) -> (element=w601:dbl[])  [unwired: 1 in]
                      n224 = Compound Arithmetic op=MULTIPLY(w601, w601, w601) -> (w603:dbl[])
                      n225 = call-poly <vilib>:"Mean.vi"("X"=w603) -> ("mean"=w602:dbl)  [unwired: 1 out]
                    }
                    frame "Pulsed Wire" {
                    }
                  }
                }
                frame True {
                  n226 = global read "Calib_global.vi" "ADAM Channel Name Vel Ref"() -> (w607:string)
                  n227 = call "Get_ref_inst_value.vi"("Ref Instrument type"=w611, "ADAM Channel Name"=w607, "Index in"=w609, "Start time"=w612) -> ("Ref Value"=w610:dbl, "Index out"=w608:i32)  [unwired: 4 in, 6 out]
                }
              }
              n228 = Build Array (concatenate)(w585, w588) -> (w584:dbl[])
            }
            frame #6 {
              n229 = case shown="\"Fast FID\"" w615 {
                tunnel: w622 -> [w627 w637 w644 w652 w664 w675]
                tunnel: [w628 w638 w645 w653 w665 w676] -> w621
                tunnel: w619 -> [w626 w636 w643 w648 w663 w674]
                tunnel: [w626 w635 w642 w646 w662 w673] -> w620
                tunnel: w618 -> [w624 _ _ w650 w658 w669]
                tunnel: w617 -> [w629 w639 _ w654 w656 w667]
                tunnel: w616 -> [_ w634 _ _ _ _]
                tunnel: w614 -> [_ _ w641 _ _ _]
                tunnel: w613 -> [_ _ w640 _ _ _]
                frame "Propeller anemometer", Default {
                  n230 = Index Array(array=w624, index=w629) -> (element=w625:T16)
                  n231 = Unbundle By Name(w625) -> ("U"=w623:dbl)
                  n232 = Build Array (concatenate)(w627, w623) -> (w628:dbl[])
                }
                frame "Generic Polynomial" {
                  n233 = Index Array(array=w634, index (row)=w639) -> (element=w631:dbl[])  [unwired: 1 in]
                  n234 = call-poly <vilib>:"Mean.vi"("X"=w631) -> ("mean"=w633:dbl)  [unwired: 1 out]
                  n235 = Multiply(x=w631, y=w631) -> (x*y=w630:dbl[])
                  n236 = call-poly <vilib>:"Mean.vi"("X"=w630) -> ("mean"=w632:dbl)  [unwired: 1 out]
                  n237 = Build Array (concatenate)(w637, w633) -> (w638:dbl[])
                  n238 = Build Array (concatenate)(w636, w632) -> (w635:dbl[])
                }
                frame "Pulsed Wire" {
                  n239 = Build Array (concatenate)(w644, w641) -> (w645:dbl[])
                  n240 = Build Array (concatenate)(w643, w640) -> (w642:dbl[])
                }
                frame "Fast FID" {
                  n241 = Index Array(array=w650, index=w654) -> (element=w651:T16)
                  n242 = Unbundle By Name(w651) -> ("U"=w649:dbl, "u^2"=w647:dbl)
                  n243 = Build Array (concatenate)(w652, w649) -> (w653:dbl[])
                  n244 = Build Array (concatenate)(w648, w647) -> (w646:dbl[])
                }
                frame "Cross wire velocity" {
                  n245 = Increment(x=w656) -> (x+1=w655:i32)
                  n246 = Index Array(array=w658, index=w656) -> (element=w661:T16)
                  n247 = Index Array(array=w658, index=w655) -> (element=w660:T16)
                  n248 = Unbundle By Name(w661) -> ("U"=w657:dbl)
                  n249 = Unbundle By Name(w660) -> ("U"=w659:dbl)
                  n250 = Build Array (concatenate)(w664, w657) -> (w665:dbl[])
                  n251 = Build Array (concatenate)(w663, w659) -> (w662:dbl[])
                }
                frame "Cross wire angle" {
                  n252 = Increment(x=w667) -> (x+1=w666:i32)
                  n253 = Index Array(array=w669, index=w667) -> (element=w672:T16)
                  n254 = Index Array(array=w669, index=w666) -> (element=w671:T16)
                  n255 = Unbundle By Name(w672) -> ("U"=w668:dbl)
                  n256 = Unbundle By Name(w671) -> ("U"=w670:dbl)
                  n257 = Build Array (concatenate)(w675, w668) -> (w676:dbl[])
                  n258 = Build Array (concatenate)(w674, w670) -> (w673:dbl[])
                }
              }
            }
            frame #7 {
              w677 = FALSE  # Visible
              n259 = global read "Meas_global.vi" "Raw data file"() -> (w679:path)
              n260 = Strip Path(path=w679) -> (stripped path=w678:path)  [unwired: 1 out]
              n261 = global write "Calib_global.vi" "Calib Raw Data Folder"(w678) -> ()
              n262 = property on="String" class="Str"("Visible"=w677, "Blinking"=w677) -> ()  [unwired: 2 in, 2 out]
            }
          }
        }
        frame "Refit Curve" {
          # "Another calibration point is not required. Also  checks if there are any points to fit curve to."
        }
      }
      "Status Out" <- w481
    }
    frame #12 {
      n263 = Build Array(w690, w693, w692, w687, w691) -> (w689:dbl[][])
      n264 = call "Sort_Array_Indicies.vi"("unsorted array"=w690) -> ("Sort Index"=w686:i32[])  [unwired: 1 out]
      n265 = for {
        tunnel: w686 -> [w696]
        tunnel: w689 -> [w695] mode=indexing
        tunnel: [w694] -> w688 mode=indexing
        n266 = for {
          tunnel: w696 -> [w699] mode=indexing
          tunnel: w695 -> [w698]
          tunnel: [w697] -> w694 mode=indexing
          n267 = Index Array(array=w698, index=w699) -> (element=w697:dbl)
        }
      }
      "Ref velocity" <- w687
    }
    frame #13 {
      w707 = FALSE  # t/f
      w708 = FALSE  # t/f
      n268 = Index Array(array="Point selector 4", index=0) -> (element=w705:cluster{"Y":dbl, "Y2":dbl, "X":dbl, "t/f":bool})
      n269 = Index Array(array="Point selector 3", index=0) -> (element=w713:cluster{"Y":dbl, "X":dbl, "t/f":bool})
      n270 = Bundle By Name(cluster=w705, "t/f"=w707) -> (w706:cluster{"Y":dbl, "Y2":dbl, "X":dbl, "t/f":bool})
      n271 = Bundle By Name(cluster=w713, "t/f"=w708) -> (w709:cluster{"Y":dbl, "X":dbl, "t/f":bool})
      n272 = Build Array (concatenate)("Point selector 4", w706) -> (w702:T5)
      n273 = Build Array (concatenate)("Point selector 3", w709) -> (w711:cluster{"Y":dbl, "X":dbl, "t/f":bool}[])
      n274 = for {
        tunnel: w711 -> [w729]
        tunnel: w715 -> [w726] mode=indexing
        tunnel: [w728] -> w712 mode=indexing
        tunnel: w702 -> [w727]
        tunnel: [w725] -> w701 mode=indexing
        n275 = Index Array(array=w729, index=w726) -> (element=w728:cluster{"Y":dbl, "X":dbl, "t/f":bool})
        n276 = Index Array(array=w727, index=w726) -> (element=w725:cluster{"Y":dbl, "Y2":dbl, "X":dbl, "t/f":bool})
      }
      n277 = call "Calib_Analyse_fit.vi"("Calib file"=w716, "Input points"=w700, "polynomial order"="polynomial order", "Fixed n"="Fixed n", "n"="n", "Point selector 3"=w712, "Point selector 4"=w701) -> ("Calib const"=→"Calib const":string[][], "Calibration plot"=→"Calibration plot":cluster{cluster{dbl, dbl}[]}[], "Point selector 3 out"=w722:cluster{"Y":dbl, "X":dbl, "t/f":bool}[], "Coefficients"=→"Coefficients":dbl[][], "Point selector 4 out"=w721:T5)  [unwired: 4 out]
      n278 = local write "Point selector 3"(w722) -> ()
      n279 = local write "Point selector 4"(w721) -> ()
    }
    frame #14 {
      w745 = FALSE  # Lock File
      w747 = FALSE  # advisory dialog? (display:T)
      w748 = FALSE  # append to file? (new file:F)
      n280 = global read "Calib_global.vi" "Calib Raw Data Folder"() -> (w738:path)
      n281 = global read "Calib_global.vi" "Calib Raw Data Folder"() -> (w737:path)
      n282 = Strip Path(path=w743) -> (name=w742:string)  [unwired: 1 out]
      n283 = List Folder(path=w738) -> (filenames=w741:string[])  [unwired: 1 in, 5 out]
      n284 = Array Size(array=w741) -> (size(s)=w740:i32)
      n285 = Greater Than 0?(x=w740) -> (x > 0?=w739:bool)
      n286 = Path To String(path=w737) -> (string=w736:string)
      n287 = call "Characters_to_string.vi"("Characters to write"=w736, "Label for characters"="Calib Raw Data Folder") -> ("Output string"=w733:string)
      n288 = Concatenate Strings(w734, w733) -> (w732:string)
      n289 = global read "Calib_global.vi" "Header string"() -> (w746:string)
      n290 = call "Add_label_to_string.vi"("String to write"=w732, "File Label"="Raw data header") -> ("Output string"=w730:string)
      n291 = Concatenate Strings(w746, w730) -> (w744:string)
      n292 = case shown="True" w739 {
        tunnel: w744 -> [_ w752]
        tunnel: w742 -> [_ w751]
        tunnel: w738 -> [_ w749]
        frame False {
        }
        frame True {
          w753 = FALSE  # Lock File
          w754 = FALSE  # append to file? (new file:F)
          w755 = FALSE  # advisory dialog? (display:T)
          n293 = Build Path(base path=w749, name or relative path=w751) -> (appended path=w750:path)
          n294 = call "Write_Characters_To_File.vi"("file path (dialog if empty)"=w750, "advisory dialog? (display:T)"=w755, "character string"=w752, "append to file? (new file:F)"=w754, "Lock File"=w753) -> ()  [unwired: 4 out]
        }
      }
      n295 = call "Write_Characters_To_File.vi"("file path (dialog if empty)"=w743, "advisory dialog? (display:T)"=w747, "character string"=w744, "append to file? (new file:F)"=w748, "Lock File"=w745) -> ()  [unwired: 4 out]
    }
    frame #15 {
      n296 = case shown="\"Take new data point\"" w758 {
        tunnel: w757 -> [w761 _]
        tunnel: w756 -> [w760 _]
        frame "Take new data point" {
          n297 = global read "Calib_global.vi" "Calib Ch No"() -> (w759:i16)
          n298 = stacked-sequence {
            tunnel: w761 -> [w762 w779]
            tunnel: w760 -> [_ w778]
            tunnel: w759 -> [w763 w772]
            frame #0 {
              n299 = Current VI's Path() -> (path=w768:path)
              n300 = call "Running_as_top_level.vi"("Vi path name"=w768) -> ("Top Level"=w767:bool)  [unwired: 1 out]
              n301 = case shown="True" w767 {
                frame False {
                }
                frame True {
                  n302 = call "Measurement.vi"("setup"=Setup."Setup Front Panel", "Post Process"=Post_Process."Take New Data", "File"=Save_Data."Save No Data") -> ()  [unwired: 4 in, 13 out]
                }
              }
              n303 = Build Array(w762) -> (w766:path[])
              n304 = Build Array(w763) -> (w765:i16[])
              n305 = call "Current_Calib_Filenames.vi"("Calib Filename"=w766, "Channel Numbers"=w765, "Mode"=App_Global."Write to Global") -> ()  [unwired: 3 out]
            }
            frame #1 {
              n306 = global read "Calib_global.vi" "Instrument type"() -> (w781:T13)
              n307 = case shown="\"Cross wire velocity\"" w781 {
                tunnel: w772 -> [_ w793 w799]
                tunnel: [path "" ("appended path") w789 w794] -> w780
                tunnel: [FALSE TRUE TRUE] -> w775
                frame "Propeller anemometer", Default {
                }
                frame "Cross wire angle" {
                  n308 = Format Into String(format string="Ch%d_XW_Angle_Calib", w793) -> (resulting string=w788:string)  [unwired: 2 in, 1 out]
                  n309 = call "Setup_Filepath.vi"("Setup File Type"=Setup_Filetype."Calibration Setups", "Filename in"=w788) -> ("Filename Out"=w789:path)  [unwired: 1 out]
                }
                frame "Cross wire velocity" {
                  n310 = Format Into String(format string="Ch%d_XW_Velocity_Calib", w799) -> (resulting string=w795:string)  [unwired: 2 in, 1 out]
                  n311 = call "Setup_Filepath.vi"("Setup File Type"=Setup_Filetype."Calibration Setups", "Filename in"=w795) -> ("Filename Out"=w794:path)  [unwired: 1 out]
                }
              }
              n312 = Array Size(array=w778) -> (size(s)=w777:i32)
              n313 = Greater?(x=w777, y=1) -> (0:w774:bool)
              n314 = And(x=w774, y=w775) -> (x .and. y?=w773:bool)
              n315 = case shown="True" w773 {
                tunnel: w780 -> [_ w784]
                tunnel: w779 -> [_ w783]
                frame False {
                }
                frame True {
                  n316 = call "Copy_with_Check.vi"("Mode"=enum16{"Move", "Copy"}."Copy", "Target Path"=w784, "Variable Target?"=FALSE, "Source Path"=w783) -> ()  [unwired: 1 out]
                }
              }
            }
          }
        }
        frame "Refit Curve" {
        }
      }
    }
    frame #16 {
      n317 = case shown="\"Take a New Calibration Point\"" w800 {
        frame "Show Setup" {
          n318 = local write "Mode"(Calib_mode."Take a New Calibration Point" ("Mode")) -> ()
        }
        frame "Take a New Calibration Point" {
        }
        frame "Refit Curve" {
        }
        frame "Setup Front Panel" {
          n319 = local write "Mode"(Calib_mode."Show Setup" ("Mode")) -> ()
        }
      }
      n320 = global write "Calib_global.vi" "Calibration Points"(dbl[] [] ("Calibration Points")) -> ()
    }
  }
